vi "Connect NetworkStream.vi"(6 "timeout (500 ms)":i32=500, 8 "error in (no error)":errorcluster, 11 "Stream Name":string) -> (0 "error out":errorcluster, 3 "Connection.NetworkStream":refnum<class "Connection.NetworkStream.lvclass">)   [LabVIEW 2013, in "Connection.NetworkQueue_GOSPL.lvlib" / "Connection.NetworkStream.lvclass"]
uses:
  Connection.NetworkStream/Connection.NetworkStream.lvclass
  Connection/Connection.lvclass
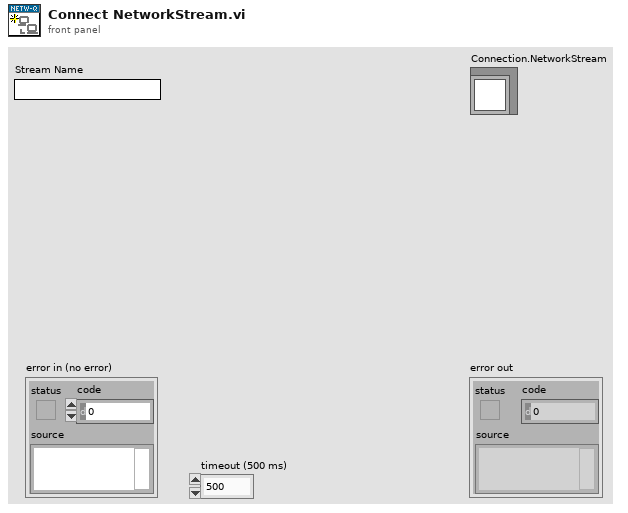
[diagram p1: front panel]
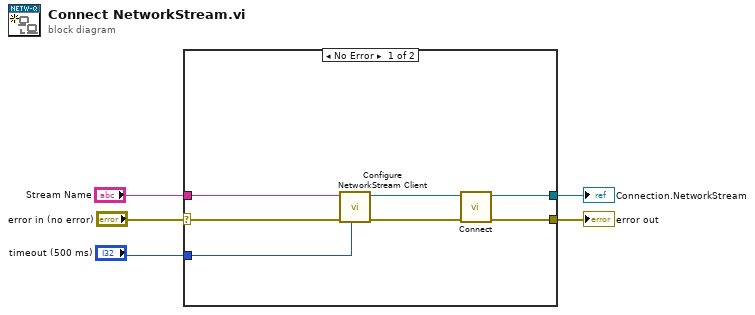
[diagram p0: block diagram]
diagram:
  n1 = case shown="No Error" "error in (no error)" {
    selector: "error in (no error)" -> [w9 w13]
    tunnel: [w11 w13] -> w4
    tunnel: [w12 _] -> w3
    tunnel: "Stream Name" -> [w7 _]
    tunnel: "timeout (500 ms)" -> [w6 _]
    frame No Error {
      n2 = call "Configure NetworkStream Client.vi"("timeout (500 ms)"=w6, "error in (no error)"=w9, "Remote URI"=w7) -> ("error out"=w8:errorcluster, "Connection.NetworkStream"=w10:refnum<class "Connection.NetworkStream.lvclass">)  [unwired: 7 in]
      n3 = call "Connect.vi"("error in (no error)"=w8, "Connection in"=w10) -> ("error out"=w11:errorcluster, "Connection out"=w12:refnum<class "Connection.NetworkStream.lvclass">)  [unwired: 7 in, 1 out]
    }
    frame Error {
    }
  }
  "error out" <- w4
  "Connection.NetworkStream" <- w3
